vi "MDAQ_ReadBuff.vi"(8 "error in":errorcluster, 11 "VISA resource name":refnum<visa-resource-name>) -> (0 "error IO":errorcluster, 1 "Buffer Not Empty":bool, 2 "read buffer":string, 3 "VISA resource name out":refnum<visa-resource-name>)   [LabVIEW 2021]
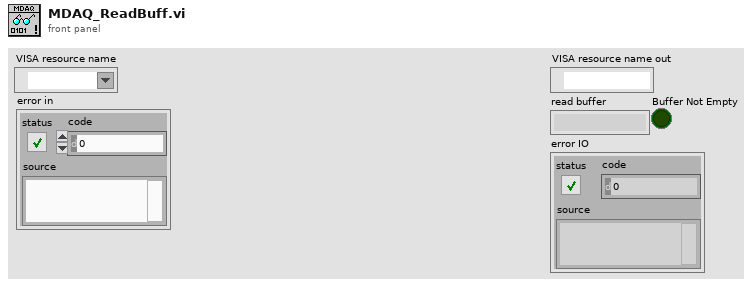
[diagram p1: front panel]
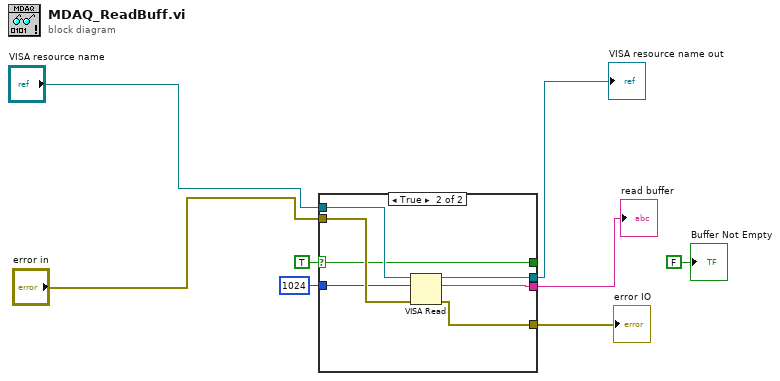
[diagram p0: block diagram]
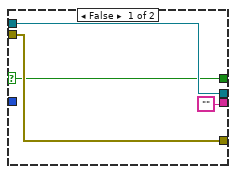
[diagram p2: hidden frame]
diagram:
  n1 = case shown="True" TRUE {
    selector: TRUE -> [w9 w13]
    tunnel: "error in" -> [w10 w19]
    tunnel: u32 1024 ("Bytes at Port") -> [_ w18]
    tunnel: [w11 w17] -> w7
    tunnel: ["" w16] -> w8
    tunnel: [w10 w15] -> w6
    tunnel: "VISA resource name" -> [w11 w14]
    tunnel: [w9 w13] -> _
    frame False {
    }
    frame True {
      n2 = VISA Read(VISA resource name=w14, byte count=w18, error in (no error)=w19) -> (VISA resource name out=w17:refnum<visa-resource-name>, read buffer=w16:string, error out=w15:errorcluster)  [unwired: 1 out]
    }
  }
  "VISA resource name out" <- w7
  "read buffer" <- w8
  "error IO" <- w6
  "Buffer Not Empty" <- FALSE ("Buffer Not Empty")
